vi "SP Save Formatting Traces.vi"(1 "LimitOn":bool, 2 "Display":T7 caption="Display (data)" items=["Data", "Memory", "Data/Memory"], 3 "Ch Index (0)":i32) -> (0 "Traces":T1[](array[typedef]))   [LabVIEW 2011]
uses:
  TypeDefs/SP Trace Types.ctl
  server/dd/lib/Report Templates/Template TDM/enumColor.ctl
  server/dd/lib/Report Templates/Template TDM/enumLineTypes.ctl
  server/dd/lib/Report Templates/Template TDM/enumLineWidths.ctl
  server/dd/lib/Report Templates/Template TDM/enumMarkerTypes.ctl
  TypeDefs/SP Trace.ctl
  TypeDefs/SP Display Data.ctl
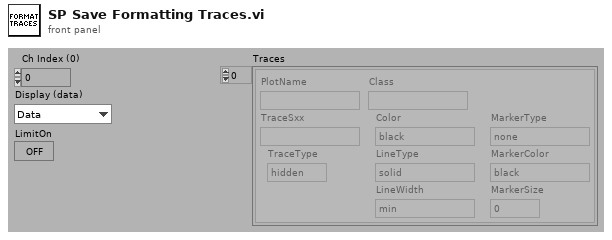
[diagram p1: front panel]
types:
  T1 = typedef "SP Trace.ctl" = cluster{"PlotName":string, "TraceSxx":string, "TraceType":T2, "Class":string, "Color":T3, "LineType":T4, "LineWidth":T5, "MarkerType":T6, "MarkerColor":T3, "MarkerSize":dbl}
  T2 = typedef "SP Trace Types.ctl" = enum16{"hidden", "data", "upper limit", "lower limit", "failures", "memory"}
  T3 = typedef "enumColor.ctl" = enum16{"black", "red", "green", "blue", "violet", "turquoise", "grey", "yell", "dark red", "dark green", "dark blue", "dark violet", "dark turquoise", "dark grey", "dark yellow", "white", "other colors", "no color"}
  T4 = typedef "enumLineTypes.ctl" = enum16{"solid", "dash&dott", "dashed 1", "dashed 2", "dotted"}
  T5 = typedef "enumLineWidths.ctl" = enum16{"min", "0.25", "0.35", "0.5", "0.7", "1.0", "1.4", "2.0", "2.8", "4.0", "5.6", "8.0", "11.2", "16.0", "22.4", "32.0"}
  T6 = typedef "enumMarkerTypes.ctl" = enum16{"none", "square", "rhomb", "triangle", "cross", "asterisk", "short dash", "long dash", "plus", "circle"}
  T7 = typedef "SP Display Data.ctl" = u16
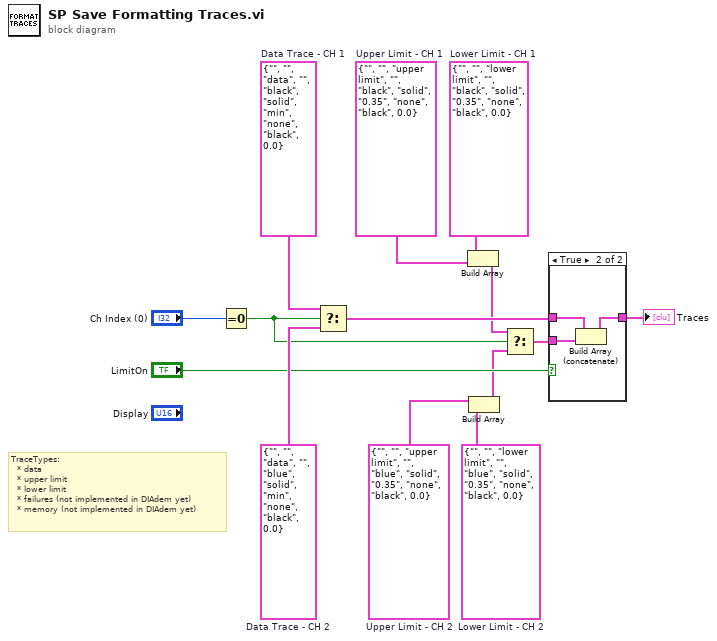
[diagram p0: block diagram]
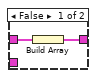
[diagram p2: hidden frame]
diagram:
  w6 = T1 {"PlotName"="", "TraceSxx"="", "TraceType"=enum."lower limit", "Class"="", "Color"=enum."blue", "LineType"=enum."solid", "LineWidth"=enum."0.35", "MarkerType"=enum."none", "MarkerColor"=enum."black", "MarkerSize"=0.0}  # Lower Limit - CH 2
  w7 = T1 {"PlotName"="", "TraceSxx"="", "TraceType"=enum."upper limit", "Class"="", "Color"=enum."blue", "LineType"=enum."solid", "LineWidth"=enum."0.35", "MarkerType"=enum."none", "MarkerColor"=enum."black", "MarkerSize"=0.0}  # Upper Limit - CH 2
  w12 = T1 {"PlotName"="", "TraceSxx"="", "TraceType"=enum."data", "Class"="", "Color"=enum."blue", "LineType"=enum."solid", "LineWidth"=enum."min", "MarkerType"=enum."none", "MarkerColor"=enum."black", "MarkerSize"=0.0}  # Data Trace - CH 2
  w9 = T1 {"PlotName"="", "TraceSxx"="", "TraceType"=enum."lower limit", "Class"="", "Color"=enum."black", "LineType"=enum."solid", "LineWidth"=enum."0.35", "MarkerType"=enum."none", "MarkerColor"=enum."black", "MarkerSize"=0.0}  # Lower Limit - CH 1
  w8 = T1 {"PlotName"="", "TraceSxx"="", "TraceType"=enum."upper limit", "Class"="", "Color"=enum."black", "LineType"=enum."solid", "LineWidth"=enum."0.35", "MarkerType"=enum."none", "MarkerColor"=enum."black", "MarkerSize"=0.0}  # Upper Limit - CH 1
  w13 = T1 {"PlotName"="", "TraceSxx"="", "TraceType"=enum."data", "Class"="", "Color"=enum."black", "LineType"=enum."solid", "LineWidth"=enum."min", "MarkerType"=enum."none", "MarkerColor"=enum."black", "MarkerSize"=0.0}  # Data Trace - CH 1
  # "TraceTypes:\n  * data\n  * upper limit\n  * lower limit\n  * failures (not implemented in DIAdem yet)\n  * memory (not implemented in DIAdem yet)"
  n1 = Equal To 0?(x="Ch Index (0)") -> (x = 0?=w5:bool)
  n2 = Select(t=w13, s=w5, f=w12) -> (s? t:f=w10:T1)
  n3 = Build Array(w9, w8) -> (w4:T1[])
  n4 = Build Array(w7, w6) -> (w3:T1[])
  n5 = Select(t=w4, s=w5, f=w3) -> (s? t:f=w2:T1[])
  n6 = case shown="True" "LimitOn" {
    tunnel: w10 -> [w16 w19]
    tunnel: w2 -> [_ w18]
    tunnel: [w15 w17] -> w1
    frame False {
      n7 = Build Array(w16) -> (w15:T1[])
    }
    frame True {
      n8 = Build Array (concatenate)(w19, w18) -> (w17:T1[])
    }
  }
  "Traces" <- w1
